vi "Last Ack.vi"(10 "Actor":refnum<class "Actor.lvclass">, 11 "jettl in":refnum<class "jettl.lvclass">) -> (3 "jettl out":refnum<class "jettl.lvclass">)   [LabVIEW 2021, in "jettl.lvlib" / "jettl.lvclass"]
uses:
  jettl.lvclass
  Actor/Actor/Actor.lvclass
  jettl.lvclass/jettl.ctl
  jettl.lvlib
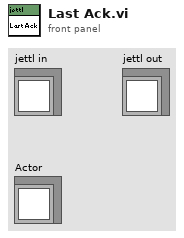
[diagram p1: front panel]
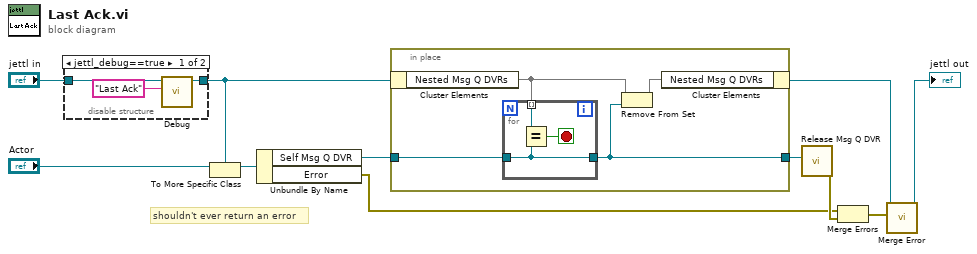
[diagram p0: block diagram]
diagram:
  # "shouldn't ever return an error"
  n1 = disable-structure shown="jettl_debug==true" {
    disable-tunnel: "jettl in" -> [w14 w15]
    disable-tunnel: [w13 w15] -> w1
    frame condition #0 (active) {
      n2 = call "Debug.vi"("Method"="Last Ack", "jettl in"=w14) -> ("jettl out"=w13:refnum<class "jettl.lvclass">)  [unwired: 9 in]
    }
    frame condition #1 {
    }
  }
  n3 = To More Specific Class(target class=w1, reference="Actor") -> (specific class reference=w11:refnum<class "jettl.lvclass">)  [unwired: 1 in, 1 out]
  n4 = Unbundle By Name(w11) -> ("Self Msg Q DVR"=w9:refnum<data-value>, "Error"=w6:errorcluster)
  n5 = in-place {
    in-place-border: w9 -> [w17]
    in-place-border: [w16] -> w8
    n6 = in-place-cluster #1(w1) -> ("Nested Msg Q DVRs"=w19:set{refnum<data-value>})
    n7 = for {
      tunnel: w17 -> [w20]
      tunnel: w19 -> [w21] mode=indexing
      tunnel: [w20] -> w16
      stop <- w22 stop-if-true
      n8 = Equal?(x=w21, y=w20) -> (x = y?=w22:bool)
    }
    n9 = Remove From Set(10:w16, 11:w19) -> (3:w18:set{refnum<data-value>})  [unwired: 1 out]
    n10 = in-place-cluster #1("Nested Msg Q DVRs"=w18) -> (w5:refnum<class "jettl.lvclass">)
  }
  n11 = call "Release Msg Q DVR.vi"("Msg Q DVR"=w8) -> ("error out"=w7:errorcluster)  [unwired: 10 in]
  n12 = Merge Errors(w6, w7) -> (w3:errorcluster)
  n13 = call-dynamic "Merge Error.vi"("Error"=w3, "jettl in"=w5) -> ("jettl out"=→"jettl out":refnum<class "jettl.lvclass">)  [unwired: 9 in]
